vi "Initialize.vi"(8 "error in (no error)":errorcluster, 11 "View Template in":refnum<class "Logger Level.lvclass">) -> (0 "error out":errorcluster, 3 "View Template out":refnum<class "Logger Level.lvclass">)   [LabVIEW 2020, in "Logger Level.lvlib" / "Logger Level.lvclass"]
uses:
  Logger Level.lvclass
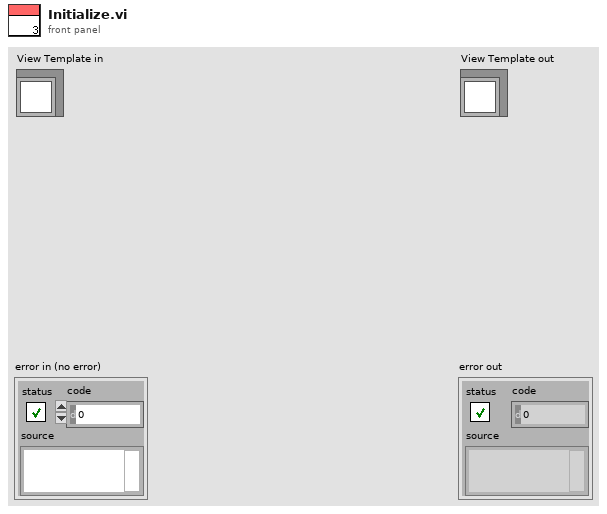
[diagram p1: front panel]
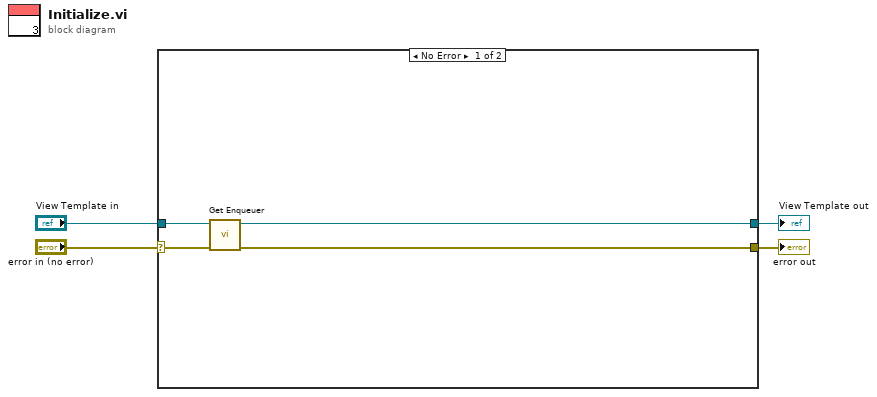
[diagram p0: block diagram]
diagram:
  n1 = case shown="No Error" "error in (no error)" {
    selector: "error in (no error)" -> [w7 w10]
    tunnel: [w5 w10] -> w3
    tunnel: [w6 w9] -> w1
    tunnel: "View Template in" -> [w8 w9]
    frame No Error {
      n2 = call "Get Enqueuer.vi"("error in (no error)"=w7, "View Template in"=w8) -> ("error out"=w5:errorcluster, "View Template out"=w6:refnum<class "Logger Level.lvclass">)  [unwired: 8 in]
    }
    frame Error {
    }
  }
  "error out" <- w3
  "View Template out" <- w1
